vi "数据全参数一起发送整点触发.vi"(6 "数据发送通道":enum16{"TCP", "VISA"}(ring), 8 "PW":string, 9 "MN":string) -> ()   [LabVIEW 2016, in "数据传输系统.lvlib"]
panel:
  out "table":string="提取小时数据"
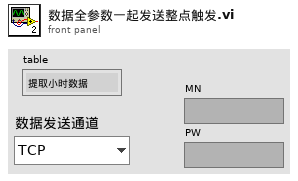
[diagram p1: front panel]
types:
  T1 = typedef "LVDateTimeRec.ctl" = cluster{"秒数的小数部分":dbl, "秒":i32, "分":i32, "时":i32, "日":i32, "月":i32, "年":i32, "天数（周）":i32, "天数（年）":i32, "DST":i32}
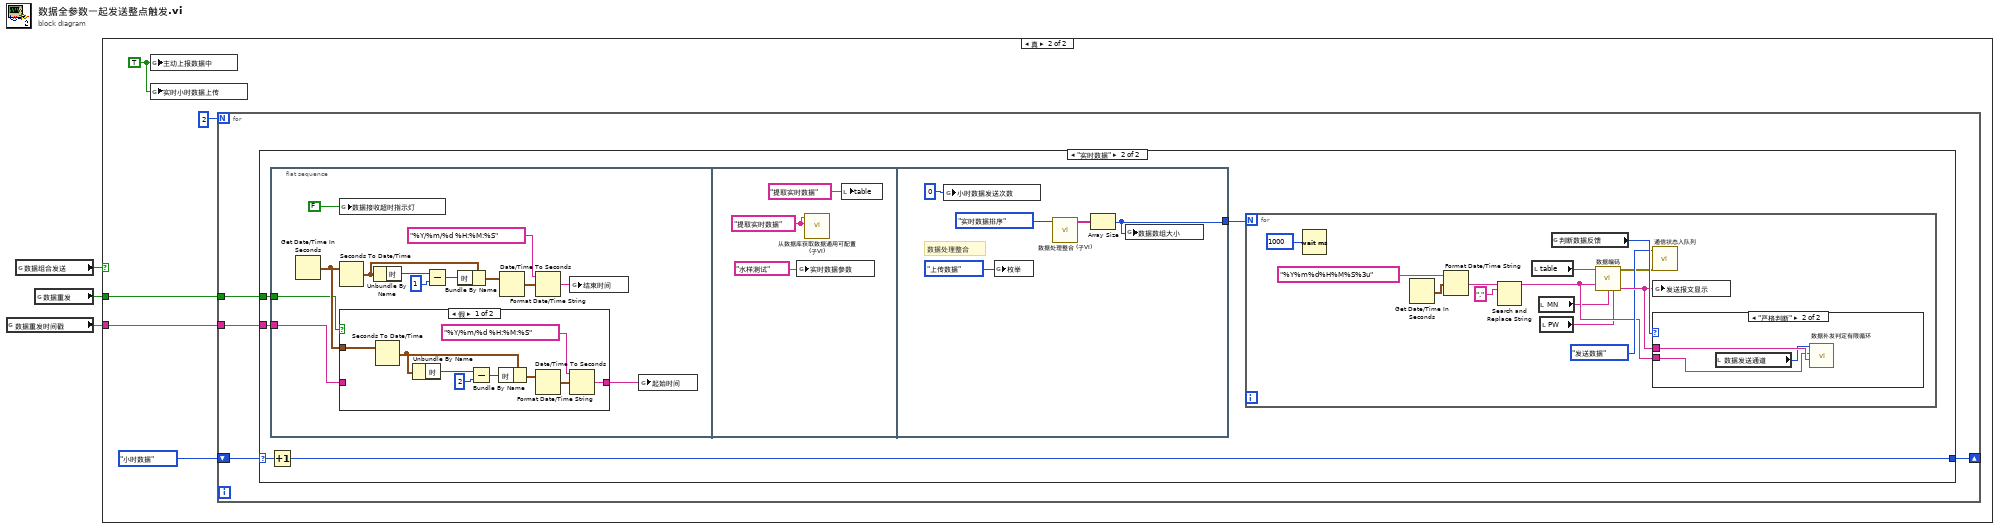
[diagram p0: block diagram]
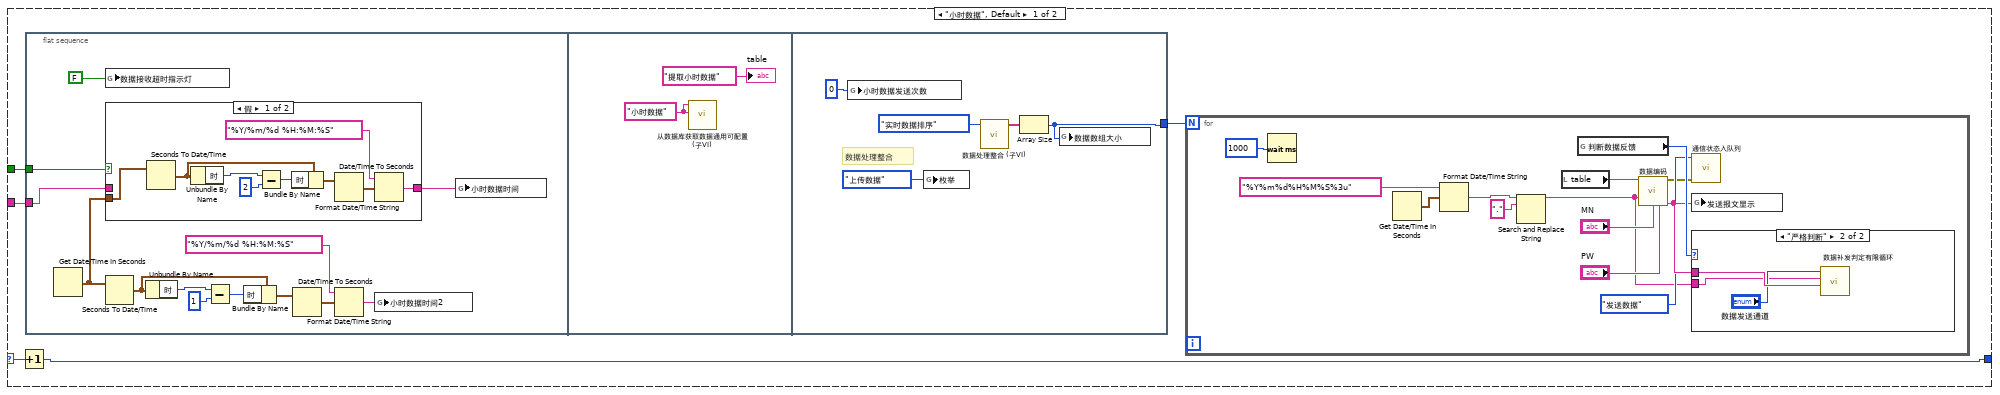
[diagram p3: hidden frame]
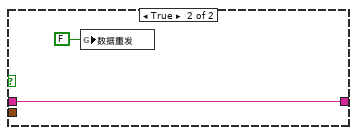
[diagram p4: hidden frame]
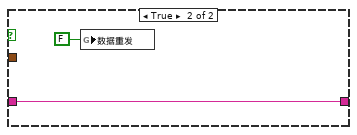
[diagram p6: hidden frame]
diagram:
  n1 = global read "断电保存全局.vi" "数据重发时间戳"() -> (w1:string)
  n2 = global read "断电保存全局.vi" "数据组合发送"() -> (w3:bool)
  n3 = global read "断电保存全局.vi" "数据重发"() -> (w2:bool)
  n4 = case shown="真" w3 {
    tunnel: w2 -> [_ w5]
    tunnel: w1 -> [_ w4]
    frame False {
    }
    frame True {
      w8 = TRUE ("主动上报数据中")
      n5 = global write "全局 数据发送重叠.vi" "主动上报数据中"(w8) -> ()
      n6 = global write "全局1.vi" "实时小时数据上传"(w8) -> ()
      n7 = for {
        N: 2 -> [_]
        shift-right: [w11] -> _
        shift-left: enum16{"小时数据", "实时数据"}."小时数据" -> [w12]
        tunnel: w5 -> [w10]
        tunnel: w4 -> [w9]
        n8 = case shown="\"实时数据\"" w12 {
          selector: w12 -> [w16 w68]
          tunnel: [w15 w67] -> w11
          tunnel: w10 -> [w14 w66]
          tunnel: w9 -> [w13 w65]
          frame "小时数据", Default {
            n9 = Increment(x=w16) -> (x+1=w15:enum16{"小时数据", "实时数据"})
            n10 = flat-sequence {
              tunnel: w14 -> [w19]
              tunnel: w13 -> [w18]
              tunnel: [w44] -> w17
              frame #0 {
                n11 = Get Date/Time In Seconds() -> (seconds since 1Jan1904=w20:timestamp)
                n12 = global write "全局 数据发送重叠.vi" "数据接收超时指示灯"(FALSE ("数据接收超时指示灯")) -> ()
                n13 = case shown="假" w19 {
                  tunnel: w20 -> [w39 _]
                  tunnel: [w31 w41] -> w23
                  tunnel: w18 -> [_ w41]
                  frame False {
                    n14 = Seconds To Date/Time(time stamp (now)=w39) -> (date time rec=w34:T1)  [unwired: 1 in]
                    n15 = Unbundle By Name(w34) -> ("时"=w32:i32)
                    n16 = Subtract(x=w32, y=2) -> (x-y=w35:i32)
                    n17 = Bundle By Name(cluster=w34, "时"=w35) -> (w36:T1)
                    n18 = Date/Time To Seconds(2:w36) -> (0:w37:timestamp)  [unwired: 1 in]
                    n19 = Format Date/Time String(time format string (%c)="%Y/%m/%d %H:%M:%S" ("时间格式字符串(%c)"), seconds (now)=w37) -> (date/time string=w31:string)  [unwired: 1 in]
                  }
                  frame True {
                    n20 = global write "断电保存全局.vi" "数据重发"(FALSE ("数据重发")) -> ()
                  }
                }
                n21 = Seconds To Date/Time(time stamp (now)=w20) -> (date time rec=w28:T1)  [unwired: 1 in]
                n22 = Unbundle By Name(w28) -> ("时"=w25:i32)
                n23 = Subtract(x=w25, y=1) -> (x-y=w27:i32)
                n24 = Bundle By Name(cluster=w28, "时"=w27) -> (w29:T1)
                n25 = Date/Time To Seconds(2:w29) -> (0:w21:timestamp)  [unwired: 1 in]
                n26 = Format Date/Time String(time format string (%c)="%Y/%m/%d %H:%M:%S" ("时间格式字符串(%c)"), seconds (now)=w21) -> (date/time string=w24:string)  [unwired: 1 in]
                n27 = global write "全局 时间2.vi" "小时数据时间2"(w24) -> ()
                n28 = global write "全局 水样时间.vi" "小时数据时间"(w23) -> ()
              }
              frame #1 {
                w43 = "小时数据" ("名称（未命名）")
                n29 = call "从数据库获取数据通用可配置(子VI).vi"("table输入"=w43, "列队名（唯一）"=w43) -> ()  [unwired: 8 in, 2 out]
                "table" <- "提取小时数据" ("新元素/子数组")
              }
              frame #2 {
                # "数据处理整合"
                n30 = global write "全局 小时数据发送次数.vi" "小时数据发送次数"(0 ("数值")) -> ()
                n31 = global write "全局1.vi" "枚举"(enum16{"返回请求应答", "上传数据", "返回执行结果"}."上传数据" ("枚举")) -> ()
                n32 = call "数据处理整合 (子VI).vi"("枚举"=enum16{"实时数据排序", "小时数据排序"}."实时数据排序") -> ("已排序的数组"=w45:string[])  [unwired: 10 in]
                n33 = Array Size(array=w45) -> (size(s)=w44:i32)
                n34 = global write "全局 数据数组大小.vi" "数据数组大小"(w44) -> ()
              }
            }
            n35 = for {
              N: w17 -> [_]
              n36 = Wait (ms)(milliseconds to wait=u32 1000 ("等待时间（毫秒）")) -> ()  [unwired: 1 out]
              n37 = Get Date/Time In Seconds() -> (seconds since 1Jan1904=w55:timestamp)
              n38 = Format Date/Time String(time format string (%c)="%Y%m%d%H%M%S%3u" ("时间格式字符串(%c)"), seconds (now)=w55) -> (date/time string=w56:string)  [unwired: 1 in]
              n39 = Search and Replace String(input string=w56, search string="." ("搜索字符串")) -> (result string=w49:string)  [unwired: 6 in, 3 out]
              n40 = local read "table"() -> (w61:string)
              n41 = global read "断电保存全局.vi" "判断数据反馈"() -> (w53:enum16{"非严格判断", "严格判断", "不判断"})
              n42 = call "数据编码.vi"("table输入"=w61, "QN"=w49, "MN"="MN", "PW"="PW") -> ("错误常量"=w50:errorcluster, "通讯包字符串"=w52:string)  [unwired: 10 in]
              n43 = call "通信状态入队列.vi"("错误输入（无错误）"=w50, "枚举"=enum16{"打开连接", "发送数据", "读取数据", "数据处理", "关闭连接"}."发送数据") -> ()  [unwired: 9 in, 1 out]
              n44 = global write "全局1.vi" "发送报文显示"(w52) -> ()
              n45 = case shown="\"严格判断\"" w53 {
                tunnel: w52 -> [_ w64]
                tunnel: w49 -> [_ w62]
                frame "非严格判断", Default {
                }
                frame "严格判断" {
                  n46 = call "数据补发判定有限循环.vi"("数据输入"=w64, "QN"=w62, "数据发送通道"="数据发送通道") -> ()  [unwired: 8 in, 1 out]
                }
              }
            }
          }
          frame "实时数据" {
            n47 = Increment(x=w68) -> (x+1=w67:enum16{"小时数据", "实时数据"})
            n48 = flat-sequence {
              tunnel: w66 -> [w73]
              tunnel: w65 -> [w72]
              tunnel: [w97] -> w69
              frame #0 {
                n49 = Get Date/Time In Seconds() -> (seconds since 1Jan1904=w74:timestamp)
                n50 = global write "全局 数据发送重叠.vi" "数据接收超时指示灯"(FALSE ("数据接收超时指示灯")) -> ()
                n51 = Seconds To Date/Time(time stamp (now)=w74) -> (date time rec=w80:T1)  [unwired: 1 in]
                n52 = case shown="假" w73 {
                  tunnel: w74 -> [w91 _]
                  tunnel: [w83 w93] -> w71
                  tunnel: w72 -> [_ w93]
                  frame False {
                    n53 = Seconds To Date/Time(time stamp (now)=w91) -> (date time rec=w86:T1)  [unwired: 1 in]
                    n54 = Unbundle By Name(w86) -> ("时"=w84:i32)
                    n55 = Subtract(x=w84, y=2) -> (x-y=w87:i32)
                    n56 = Bundle By Name(cluster=w86, "时"=w87) -> (w88:T1)
                    n57 = Date/Time To Seconds(2:w88) -> (0:w89:timestamp)  [unwired: 1 in]
                    n58 = Format Date/Time String(time format string (%c)="%Y/%m/%d %H:%M:%S" ("时间格式字符串(%c)"), seconds (now)=w89) -> (date/time string=w83:string)  [unwired: 1 in]
                  }
                  frame True {
                    n59 = global write "断电保存全局.vi" "数据重发"(FALSE ("数据重发")) -> ()
                  }
                }
                n60 = Unbundle By Name(w80) -> ("时"=w77:i32)
                n61 = Subtract(x=w77, y=1) -> (x-y=w79:i32)
                n62 = Bundle By Name(cluster=w80, "时"=w79) -> (w81:T1)
                n63 = Date/Time To Seconds(2:w81) -> (0:w75:timestamp)  [unwired: 1 in]
                n64 = Format Date/Time String(time format string (%c)="%Y/%m/%d %H:%M:%S" ("时间格式字符串(%c)"), seconds (now)=w75) -> (date/time string=w70:string)  [unwired: 1 in]
                n65 = global write "起始时间.vi" "结束时间"(w70) -> ()
                n66 = global write "起始时间.vi" "起始时间"(w71) -> ()
              }
              frame #1 {
                w96 = "提取实时数据" ("名称（未命名）")
                n67 = global write "全局 实时数据参数.vi" "实时数据参数"("水样测试" ("实时数据参数")) -> ()
                n68 = call "从数据库获取数据通用可配置(子VI).vi"("table输入"=w96, "列队名（唯一）"=w96) -> ()  [unwired: 8 in, 2 out]
                n69 = local write "table"("提取实时数据" ("新元素/子数组")) -> ()
              }
              frame #2 {
                # "数据处理整合"
                n70 = global write "全局 小时数据发送次数.vi" "小时数据发送次数"(0 ("数值")) -> ()
                n71 = global write "全局1.vi" "枚举"(enum16{"返回请求应答", "上传数据", "返回执行结果"}."上传数据" ("枚举")) -> ()
                n72 = call "数据处理整合 (子VI).vi"("枚举"=enum16{"实时数据排序", "小时数据排序"}."实时数据排序") -> ("已排序的数组"=w98:string[])  [unwired: 10 in]
                n73 = Array Size(array=w98) -> (size(s)=w97:i32)
                n74 = global write "全局 数据数组大小.vi" "数据数组大小"(w97) -> ()
              }
            }
            n75 = for {
              N: w69 -> [_]
              n76 = Wait (ms)(milliseconds to wait=u32 1000 ("等待时间（毫秒）")) -> ()  [unwired: 1 out]
              n77 = Get Date/Time In Seconds() -> (seconds since 1Jan1904=w110:timestamp)
              n78 = Format Date/Time String(time format string (%c)="%Y%m%d%H%M%S%3u" ("时间格式字符串(%c)"), seconds (now)=w110) -> (date/time string=w111:string)  [unwired: 1 in]
              n79 = Search and Replace String(input string=w111, search string="." ("搜索字符串")) -> (result string=w104:string)  [unwired: 6 in, 3 out]
              n80 = local read "table"() -> (w114:string)
              n81 = local read "MN"() -> (w103:string)
              n82 = local read "PW"() -> (w102:string)
              n83 = global read "断电保存全局.vi" "判断数据反馈"() -> (w108:enum16{"非严格判断", "严格判断", "不判断"})
              n84 = call "数据编码.vi"("table输入"=w114, "QN"=w104, "MN"=w103, "PW"=w102) -> ("错误常量"=w105:errorcluster, "通讯包字符串"=w107:string)  [unwired: 10 in]
              n85 = call "通信状态入队列.vi"("错误输入（无错误）"=w105, "枚举"=enum16{"打开连接", "发送数据", "读取数据", "数据处理", "关闭连接"}."发送数据") -> ()  [unwired: 9 in, 1 out]
              n86 = global write "全局1.vi" "发送报文显示"(w107) -> ()
              n87 = case shown="\"严格判断\"" w108 {
                tunnel: w107 -> [_ w117]
                tunnel: w104 -> [_ w116]
                frame "非严格判断", Default {
                }
                frame "严格判断" {
                  n88 = local read "数据发送通道"() -> (w115:enum16{"TCP", "VISA"})
                  n89 = call "数据补发判定有限循环.vi"("数据输入"=w117, "QN"=w116, "数据发送通道"=w115) -> ()  [unwired: 8 in, 1 out]
                }
              }
            }
          }
        }
      }
    }
  }
